vi "Choreo_TrajectorySwerve_GetTrajSample.vi"(9 "index":i32, 11 "ChoreoTrajectorySwerve":T2) -> (3 "ChoreoSwerveSample":T1)   [LabVIEW 2019, in "ChoreoLib.lvlib"]
doc: "Return a particular swerve trajectory sample\n\nInputs:\n -- ChoreoTrajectorySwerve - cluster - data cluster for this trajectory \n -- index - integer - zero relative index into the array of samples\n\nOutputs:\n -- ChoreoSwerveSample - cluster - selected trajectory sample"
uses:
  ChoreoLib.lvlib
  TypeDef/ChoreoTrajectorySwerve.ctl
  TypeDef/ChoreoSwerveSample.ctl
  TypeDef/ChoreoEventMarker.ctl
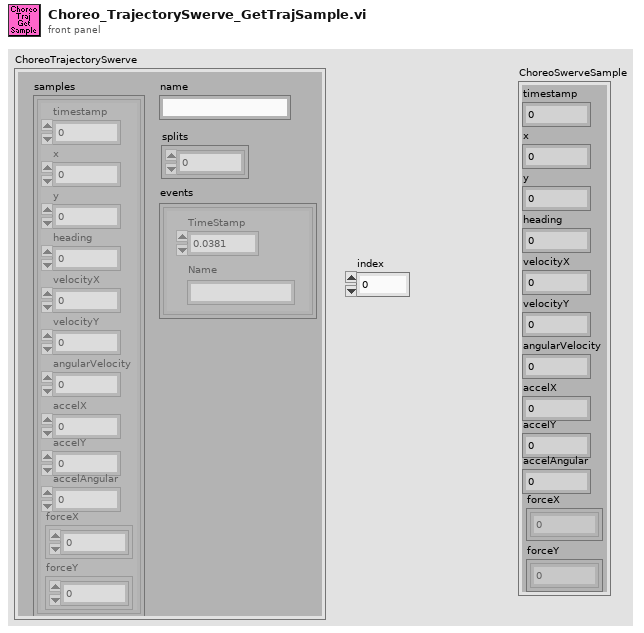
[diagram p1: front panel]
types:
  T1 = typedef "ChoreoLib.lvlib/ChoreoSwerveSample.ctl" = cluster{"timestamp":dbl, "x":dbl, "y":dbl, "heading":dbl, "velocityX":dbl, "velocityY":dbl, "angularVelocity":dbl, "accelX":dbl, "accelY":dbl, "accelAngular":dbl, "forceX":dbl[], "forceY":dbl[]}
  T2 = typedef "ChoreoLib.lvlib/ChoreoTrajectorySwerve.ctl" = cluster{"name":string, "samples":T1[], "splits":i32[], "events":T3[]}
  T3 = typedef "ChoreoLib.lvlib/ChoreoEventMarker.ctl" = cluster{"TimeStamp":dbl, "Name":string}
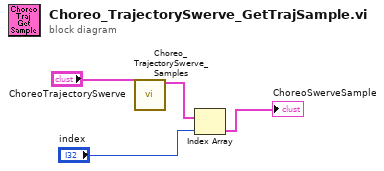
[diagram p0: block diagram]
diagram:
  n1 = call "Choreo_TrajectorySwerve_Samples.vi"("ChoreoTrajectorySwerve"="ChoreoTrajectorySwerve") -> ("samples"=w2:T1[])  [unwired: 10 in]
  n2 = Index Array(array=w2, index="index") -> (element=→"ChoreoSwerveSample":T1)
